vi "Demo Load Image.vi"() -> ()   [LabVIEW 2016]
doc: "This demo VI shows the functionality that the .NET PictureBox has when displaying images on a front panel. This VI can display any <B>Image File</B> into the PictureBox control, and then automatically control the <B>Size Mode (Zoom)</B> without any additional LabVIEW code. This demo VI also shows the opacity feature with <B>Grey Out Image?</B>, and the <B>Background Color</B>.\n\n-----\nBrian Hoover (hooovahh)"
uses:
  System.Windows.Forms
  Convert to 32Bit Image.vi
  <vilib>/Utility/colorconv.llb/Color to RGB.vi
panel:
  in  "PictureBox":refnum<k24>(container)
  out "2D Picture":picture
  in  "Grey Out Image?":bool
  in  "Size Mode (Zoom)":enum16{"Normal", "Stretch", "Center", "Zoom"}(ring)=enum."Zoom"
  in  "Background Color":u32(colorbox)=16777215
  in  "Image File":path=path "C:/My LabVIEW/Thumbnail Grid Hooovahh edit/Native Test/images/address-book-new.png"
  in  "stop":bool
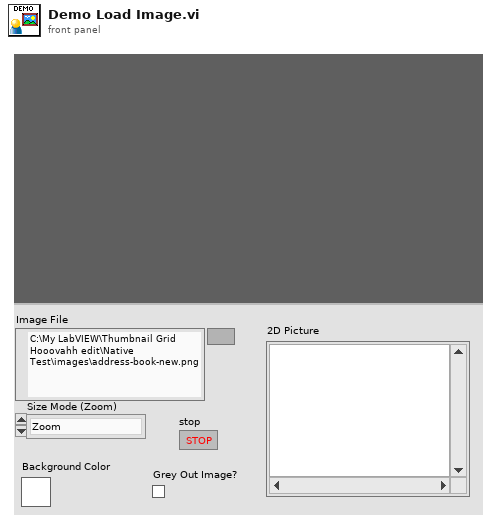
[diagram p1: front panel]
types:
  T1 = typedef "imagedata.ctl" = cluster{"image type":i32, "image depth":i32, "image":u8[], "mask":u8[], "colors":u32[], "Rectangle":cluster{"left":i16, "top":i16, "right":i16, "bottom":i16}}
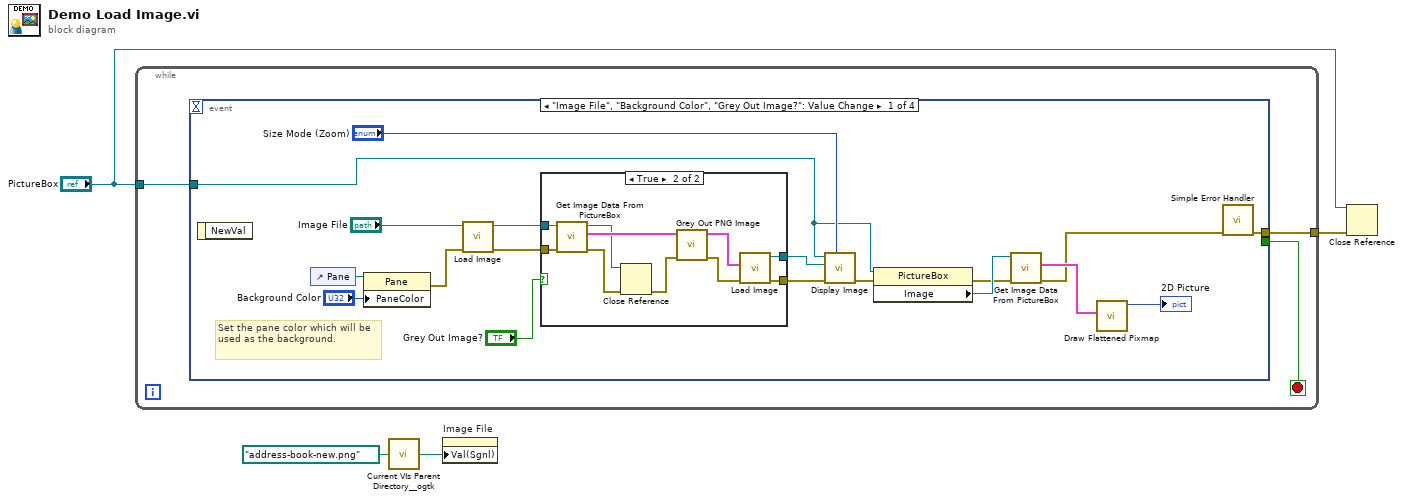
[diagram p0: block diagram]
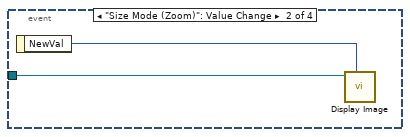
[diagram p3: hidden frame]
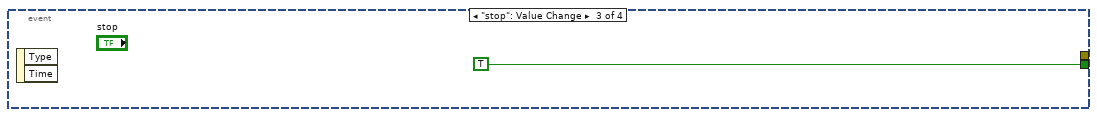
[diagram p4: hidden frame]
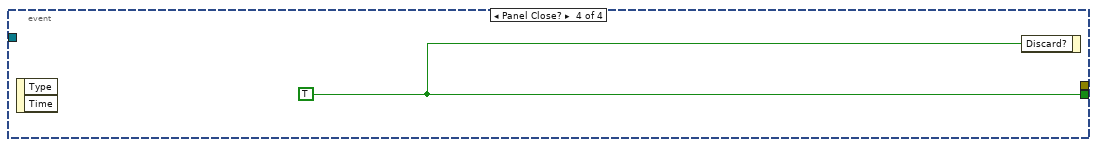
[diagram p5: hidden frame]
diagram:
  n1 = while {
    tunnel: "PictureBox" -> [w6]
    tunnel: [w5] -> w1
    stop <- w7 stop-if-true
    n2 = event shown="[0] \"Image File\", \"Background Color\", \"Grey Out Image?\": Value Change" {
      selector: _ -> [_ _ _ _]
      dyn-events: _ -> [_ _ _ _]
      timeout: _ -> [_ _ _ _]
      tunnel: [_ _ TRUE w41] -> w7
      tunnel: w6 -> [w13 w38 _ _]
      tunnel: [w18 _ _ _] -> w5
      event "Image File", "Background Color", "Grey Out Image?": Value Change {
        # "Set the pane color which will be used as the background."
        n3 = event-data() -> ()  [unwired: 1 in, 1 out]
        n4 = control-ref of="Pane"() -> (w25:refnum<vi>)
        n5 = property class="Pane"(reference=w25, "PaneColor"="Background Color") -> (error out=w23:errorcluster)  [unwired: 1 in, 1 out]
        n6 = call "Load Image.vi"("error in (no error)"=w23, "Image File"="Image File") -> ("error out"=w16:errorcluster, "Image"=w17:refnum<k24>)  [unwired: 8 in]
        n7 = case shown="True" "Grey Out Image?" {
          tunnel: [w27 w32] -> w21
          tunnel: [w26 w31] -> w19
          tunnel: w17 -> [w27 w30]
          tunnel: w16 -> [w26 w29]
          frame False {
          }
          frame True {
            n8 = call "Get Image Data From PictureBox.vi"("error in (no error)"=w29, "Image"=w30) -> ("error out"=w34:errorcluster, "Image Data"=w37:T1, "Image Out"=w35:refnum<k24>)  [unwired: 7 in]
            n9 = Close Reference(reference=w35, error in (no error)=w34) -> (error out=w33:errorcluster)
            n10 = call "Grey Out PNG Image.vi"("error in (no error)"=w33, "Image Data in"=w37) -> ("error out"=w36:errorcluster, "Image Data out"=w28:T1)  [unwired: 8 in]
            n11 = call "Load Image.vi"("error in (no error)"=w36, "Image Data"=w28) -> ("error out"=w31:errorcluster, "Image"=w32:refnum<k24>)  [unwired: 8 in]
          }
        }
        n12 = call "Display Image.vi"("Size Mode (Zoom)"="Size Mode (Zoom)", "error in (no error)"=w19, "Image"=w21, "PictureBox"=w13) -> ("error out"=w14:errorcluster)  [unwired: 6 in, 1 out]
        n13 = property class="PictureBox"(reference=w13, error in=w14) -> (error out=w11:errorcluster, "Image"=w12:refnum<k24>)  [unwired: 1 out]
        n14 = call "Get Image Data From PictureBox.vi"("error in (no error)"=w11, "Image"=w12) -> ("error out"=w8:errorcluster, "Image Data"=w10:T1)  [unwired: 7 in, 1 out]
        n15 = call <vilib>:"Draw Flattened Pixmap.vi"("image data"=w10) -> ("new picture"=→"2D Picture":picture)  [unwired: 8 in]
        n16 = call <vilib>:"Simple Error Handler.vi"("error in (no error)"=w8) -> ("error out"=w18:errorcluster)  [unwired: 4 in, 4 out]
      }
      event "Size Mode (Zoom)": Value Change {
        n17 = event-data() -> ("NewVal"=w39:enum16{"Normal", "Stretch", "Center", "Zoom"})  [unwired: 1 in]
        n18 = call "Display Image.vi"("Size Mode (Zoom)"=w39, "PictureBox"=w38) -> ()  [unwired: 8 in, 2 out]
      }
      event "stop": Value Change {
        n19 = event-data() -> ()  [unwired: 1 in, 2 out]
      }
      event Panel Close? {
        w41 = TRUE
        n20 = event-data() -> ()  [unwired: 1 in, 2 out]
        n21 = event-data("Discard?"=w41) -> ()  [unwired: 1 in, 1 out]
      }
    }
  }
  n22 = call <userlib>:"Current VIs Parent Directory__ogtk.vi"("Relative path (.)"=path "address-book-new.png") -> ("Parent Directory (+ Relative)"=w3:path)  [unwired: 4 in]
  n23 = property on="Image File" class="Path"("Val(Sgnl)"=w3) -> ()  [unwired: 2 in, 2 out]
  n24 = Close Reference(reference="PictureBox", error in (no error)=w1) -> ()  [unwired: 1 out]
